vi "addDelayTicks.vi"(8 "error in (no error)":errorcluster, 10 "Ticks":u16, 11 "Subnet in":refnum<class "Subnet.lvclass">) -> (0 "error out":errorcluster, 3 "Subnet out":refnum<class "Subnet.lvclass">)   [LabVIEW 2016]
uses:
  Common_RT_Modbus/IModbus/IModbus.lvclass
  Subnet.lvclass
  D:/Code/ts_modbus/RT/ISubnet/ISubnet.lvclass
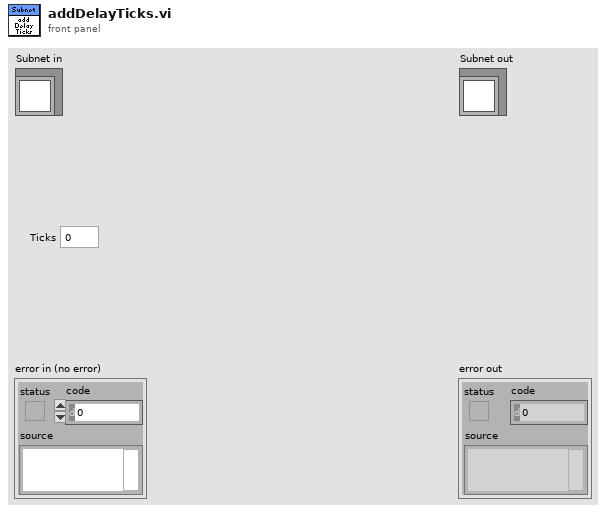
[diagram p1: front panel]
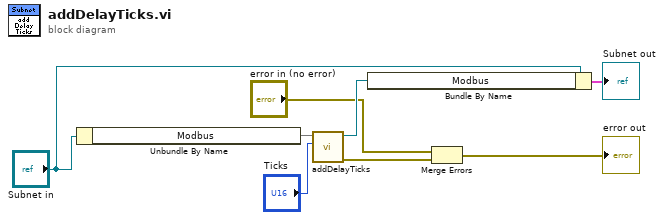
[diagram p0: block diagram]
diagram:
  n1 = Unbundle By Name("Subnet in") -> ("Modbus"=w6)
  n2 = call-dynamic "addDelayTicks.vi"("Ticks"="Ticks", "IModbus in"=w6) -> ("error out"=w3:errorcluster, "IModbus out"=w5:refnum<class "IModbus.lvclass">)  [unwired: 8 in]
  n3 = Bundle By Name(cluster="Subnet in", "Modbus"=w5) -> (→"Subnet out":cluster{})
  n4 = Merge Errors("error in (no error)", w3) -> (→"error out":errorcluster)
